vi "SI LIB Recursive File List.vi"(4 "Error in":errorcluster, 5 "Pattern (*.*)":string="*.*", 7 "Start Path\n(empty - Prompt)":path) -> (0 "Error out":errorcluster, 3 "Files":path[](array[path]))   [LabVIEW 2011]
doc: "This VI searches for all the VIs in the hierarchy of a given VI and returns an array of their paths. \nEach VI is returned once in the list, regardless of how may times it appears in the hierarchy."
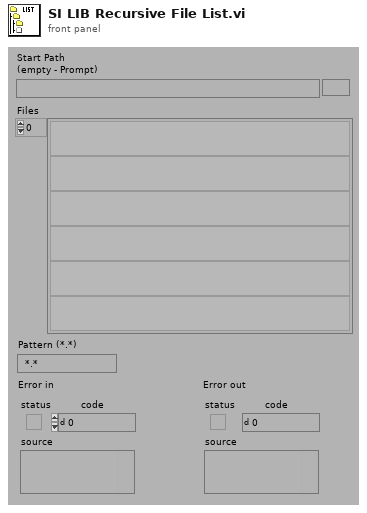
[diagram p1: front panel]
types:
  T1 = enum32{"existing file", "new file", "new or existing file", "existing dir", "new dir", "new or existing dir", "existing file (use LLBs)", "new file (use LLBs)", "new or existing file (use LLBs)", "new or existing file or directory (use LLBs)"}
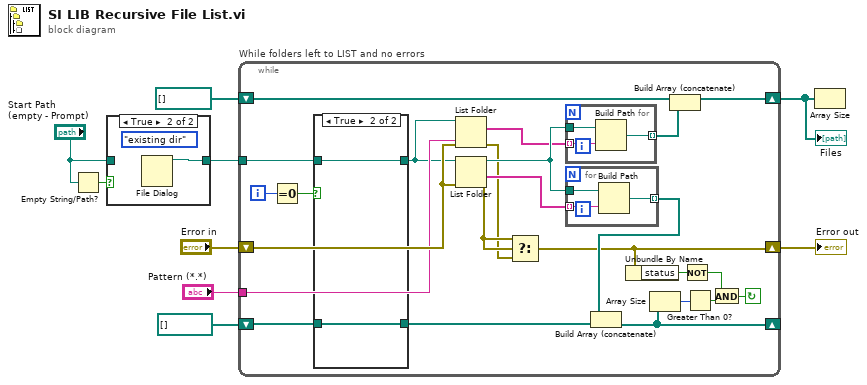
[diagram p0: block diagram]
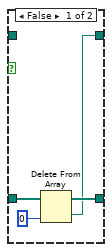
[diagram p2: hidden frame]
diagram:
  n1 = Empty String/Path?(string/path="Start Path\n(empty - Prompt)") -> (empty?=w6:bool)
  n2 = case shown="True" w6 {
    tunnel: "Start Path\n(empty - Prompt)" -> [w10 _]
    tunnel: [w10 w11] -> w4
    frame False {
    }
    frame True {
      (unwired) T1."existing dir" ("select mode (2)")
      n3 = File Dialog() -> (3:w11:path)  [unwired: 1 in, 9 out]
    }
  }
  n4 = while "While folders left to LIST and no errors" {
    tunnel: w4 -> [w30]
    shift-left: path[] [] -> [w29]
    shift-right: [w26] -> _
    shift-left: path[] [] -> [w35]
    shift-right: [w34] -> w8
    shift-left: "Error in" -> [w18]
    shift-right: [w12] -> w3
    tunnel: "Pattern (*.*)" -> [w17]
    i -> [w32]
    stop <- w27 continue-if-true
    n5 = Equal To 0?(x=w32) -> (x = 0?=w31:bool)
    n6 = case shown="True" w31 {
      tunnel: [w39 w43] -> w16
      tunnel: w30 -> [_ w43]
      tunnel: w29 -> [w42 w44]
      tunnel: [w41 w44] -> w28
      frame False {
        n7 = Delete From Array(array=w42, index=0 ("Index")) -> (deleted portion=w39:path, array with subset deleted=w41:path[])  [unwired: 1 in]
      }
      frame True {
      }
    }
    n8 = List Folder(path=w16, pattern=w17, error in=w18) -> (filenames=w15:string[], error out=w13:errorcluster)  [unwired: 3 out]
    n9 = List Folder(path=w16, error in=w18) -> (path out=w21:path, folder names=w20:string[], error out=w14:errorcluster)  [unwired: 3 out]
    n10 = Select(t=w14, s=w14, f=w13) -> (s? t:f=w12:errorcluster)
    n11 = for {
      tunnel: w15 -> [w47] mode=indexing
      tunnel: w21 -> [w46]
      tunnel: [w45] -> w33 mode=indexing
      n12 = Build Path(base path=w46, name or relative path=w47) -> (appended path=w45:path)
    }
    n13 = for {
      tunnel: w21 -> [w38]
      tunnel: w20 -> [w37] mode=indexing
      tunnel: [w36] -> w19 mode=indexing
      n14 = Build Path(base path=w38, name or relative path=w37) -> (appended path=w36:path)
    }
    n15 = Build Array (concatenate)(w19, w28) -> (w26:path[])
    n16 = Unbundle By Name(w12) -> ("status"=w23:bool)
    n17 = Array Size(array=w26) -> (size(s)=w25:i32)
    n18 = Build Array (concatenate)(w35, w33) -> (w34:path[])
    n19 = Not(x=w23) -> (.not. x?=w22:bool)
    n20 = Greater Than 0?(x=w25) -> (x > 0?=w24:bool)
    n21 = And(x=w22, y=w24) -> (x .and. y?=w27:bool)
  }
  "Error out" <- w3
  "Files" <- w8
  n22 = Array Size(array=w8) -> ()  [unwired: 1 out]
